vi "initialize.vi"(8 "error in (no error)":errorcluster, 11 "DomeController in":refnum<class "DomeController.lvclass">) -> (0 "error out":errorcluster, 3 "DomeController out":refnum<class "DomeController.lvclass">)   [LabVIEW 2016, in "DomeController.lvclass"]
uses:
  DomeController.lvclass
  DomeController.lvclass/DomeController.ctl
  domeCommunicator/DomeCommunicator.lvclass
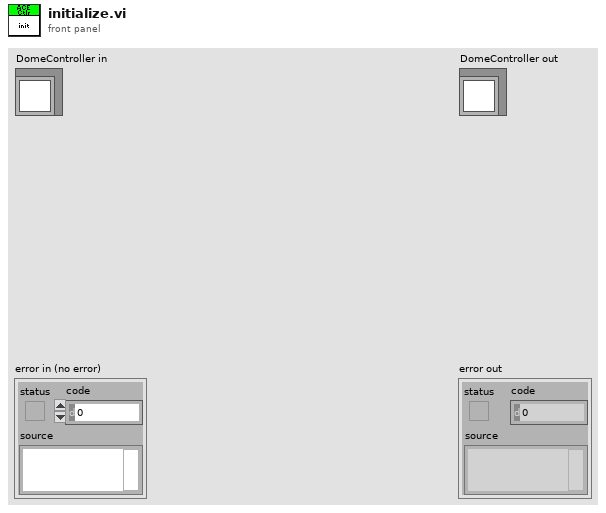
[diagram p1: front panel]
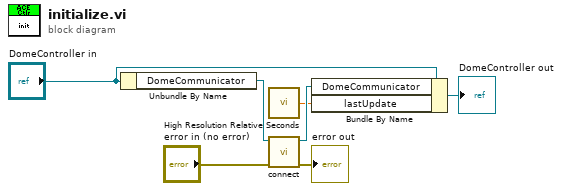
[diagram p0: block diagram]
diagram:
  n1 = Unbundle By Name("DomeController in") -> ("DomeCommunicator"=w7:refnum<class "DomeCommunicator.lvclass">)
  n2 = call <vilib>:"High Resolution Relative Seconds.vi"() -> ("relative seconds"=w1:dbl)
  n3 = call-dynamic "connect.vi"("error in (no error)"="error in (no error)", "tcpDevice in"=w7) -> ("error out"=→"error out":errorcluster, "tcpDevice out"=w3:refnum<class "DomeCommunicator.lvclass">)  [unwired: 8 in]
  n4 = Bundle By Name(cluster="DomeController in", "DomeCommunicator"=w3, "lastUpdate"=w1) -> (→"DomeController out":refnum<class "DomeController.lvclass">)
